vi "Servo (Bob).vi"(11 "Ângulo Servo:":dbl) -> ()   [LabVIEW 2013]
uses:
  <vilib>/LabVIEW Interface for Arduino/LabVIEW Interface for Arduino.lvlib
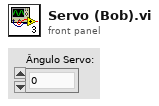
[diagram p1: front panel]
types:
  T1 = typedef "LabVIEW Interface for Arduino.lvlib/Arduino Resource.ctl" = cluster{"VISA resource":refnum<visa-resource-name>, "Board Type":T2, "Connection Type":enum8{"USB / Serial"}, "Bytes Per Packet (15)":u8}
  T2 = typedef "LabVIEW Interface for Arduino.lvlib/Board Type.ctl" = enum16{"Uno", "Dimuelanove w/Atmega 328", "Mega 2560"}
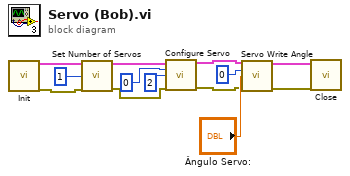
[diagram p0: block diagram]
diagram:
  n1 = call <vilib>:"Init.vi"() -> ("Arduino Resource"=w13:T1, "error out"=w9:errorcluster)  [unwired: 18 in]
  n2 = call <vilib>:"Set Number of Servos.vi"("Arduino Resource"=w13, "Number Of Servos (1)"=1, "error in"=w9) -> ("Arduino Resource"=w7:T1, "error out"=w5:errorcluster)  [unwired: 11 in]
  n3 = call <vilib>:"Configure Servo.vi"("Arduino Resource"=w7, "Servo Number (0)"=0, "DIO Pin (2)"=2, "error in"=w5) -> ("Arduino Resource"=w4:T1, "error out"=w3:errorcluster)  [unwired: 10 in]
  n4 = call <vilib>:"Servo Write Angle.vi"("Arduino Resource"=w4, "Servo Number"=0, "Angle (Degrees)"="Ângulo Servo:", "error in"=w3) -> ("Arduino Resource"=w2:T1, "error out"=w1:errorcluster)  [unwired: 10 in]
  n5 = call <vilib>:"Close.vi"("Arduino Resource"=w2, "error in"=w1) -> ()  [unwired: 13 in, 1 out]
